vi "Save RAW data.vi"(5 "Test label":string, 6 "Notes":string, 7 "User":string, 8 "Error In":errorcluster, 9 "YPR data":cluster{"Yaw":sgl, "Pitch":sgl, "Roll":sgl}[](array[cluster]), 10 "Strain data":T1(array[cluster])) -> (0 "Error Out":errorcluster)   [LabVIEW 2016]
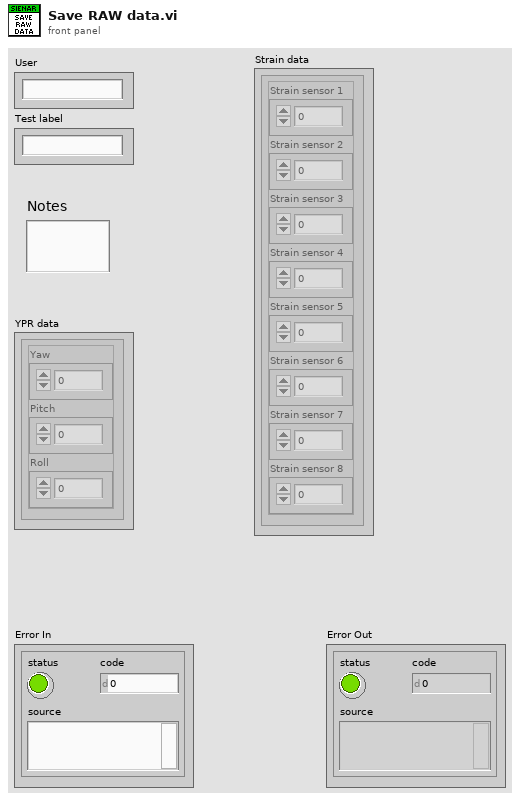
[diagram p1: front panel]
types:
  T1 = cluster{"Strain sensor 1":sgl, "Strain sensor 2":sgl, "Strain sensor 3":sgl, "Strain sensor 4":sgl, "Strain sensor 5":sgl, "Strain sensor 6":sgl, "Strain sensor 7":sgl, "Strain sensor 8":sgl}[]
  T2 = enum16{"open", "open or create", "create or replace", "create", "open (read-only)"}
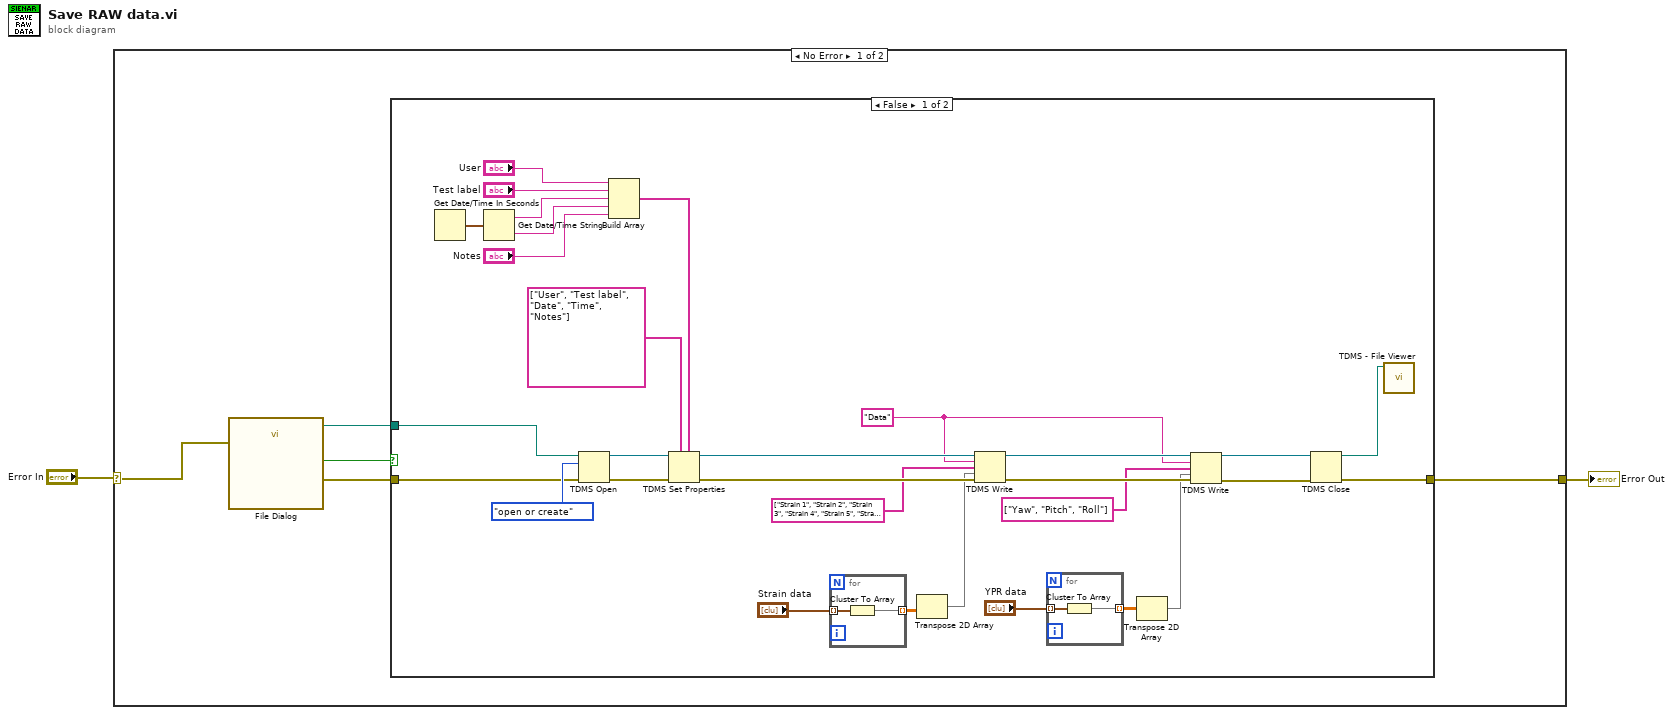
[diagram p0: block diagram]
diagram:
  n1 = case shown="No Error" "Error In" {
    selector: "Error In" -> [w5 w43]
    tunnel: [w6 w43] -> w1
    frame No Error {
      n2 = call "File Dialog"("error in"=w5) -> ("selected path"=w7:path, "cancelled"=w3:bool, "error out"=w4:errorcluster)  [unwired: 11 in, 1 out]
      n3 = case shown="False" w3 {
        tunnel: w7 -> [w27 _]
        tunnel: [w25 w42] -> w6
        tunnel: w4 -> [w26 w42]
        frame False {
          w16 = "Data" ("group name in (Untitled)")
          n4 = Get Date/Time In Seconds() -> (seconds since 1Jan1904=w31:timestamp)
          n5 = Get Date/Time String(seconds (now)=w31) -> (date string=w32:string, time string=w30:string)  [unwired: 2 in]
          n6 = TDMS Open(8:w26, 10:T2."open or create" ("operation (0:open)"), 11:w27) -> (0:w36:errorcluster, 3:w35:refnum<k34>)  [unwired: 4 in]
          n7 = Build Array("User", "Test label", w32, w30, "Notes") -> (w29:string[])
          n8 = TDMS Set Properties(5:w29, 7:string[] ["User", "Test label", "Date", "Time", "Notes"], 8:w36, 11:w35) -> (0:w23:errorcluster, 3:w22:refnum<k34>)  [unwired: 2 in, 2 out]
          n9 = for {
            tunnel: "Strain data" -> [w39] mode=indexing
            tunnel: [w38] -> w11 mode=indexing
            n10 = Cluster To Array(cluster=w39) -> (array=w38:sgl[])
          }
          n11 = Transpose 2D Array(2D array=w11) -> (transposed array=w10:sgl[][])
          n12 = TDMS Write(0:w22, 5:w16, 7:string[] ["Strain 1", "Strain 2", "Strain 3", "Strain 4", "Strain 5", "Strain 6", "Strain 7", "Strain 8"], 9:w10, 11:w23) -> (4:w24:refnum<k34>, 15:w19:errorcluster)  [unwired: 1 in, 2 out]
          n13 = for {
            tunnel: "YPR data" -> [w41] mode=indexing
            tunnel: [w40] -> w13 mode=indexing
            n14 = Cluster To Array(cluster=w41) -> (array=w40:sgl[])
          }
          n15 = Transpose 2D Array(2D array=w13) -> (transposed array=w9:sgl[][])
          n16 = TDMS Write(0:w24, 5:w16, 7:string[] ["Yaw", "Pitch", "Roll"], 9:w9, 11:w19) -> (4:w20:refnum<k34>, 15:w18:errorcluster)  [unwired: 1 in, 2 out]
          n17 = TDMS Close(8:w18, 11:w20) -> (0:w25:errorcluster, 3:w15:path)
          n18 = call <vilib>:"TDMS - File Viewer.vi"("file path"=w15) -> ()  [unwired: 5 in, 2 out]
        }
        frame True {
        }
      }
    }
    frame Error {
    }
  }
  "Error Out" <- w1
